vi "FL_Last_N_Samples_Cluster.vi"(1 "BufferLengthSamples":u32=20, 2 "Input cluster":T1) -> (0 "Output 1D array of clusters":cluster{"X":dbl, "Y":dbl}[](array[cluster]))   [LabVIEW 2016]
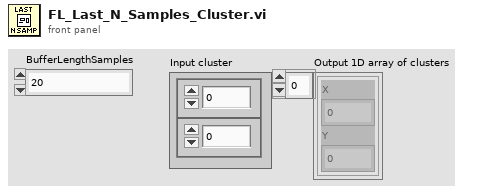
[diagram p1: front panel]
types:
  T1 = cluster{"Numeric Control":dbl, "Numeric Control":dbl}
  T2 = cluster{"Numeric Control":dbl, "Numeric Control":dbl}[]
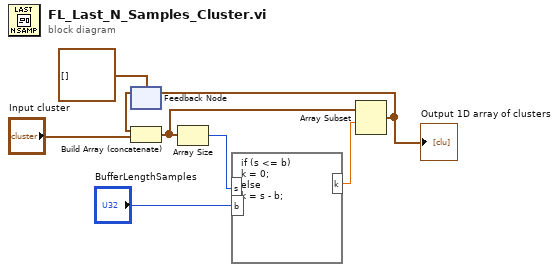
[diagram p0: block diagram]
diagram:
  n1 = feedback #1(T2 []) -> (w6:T2)
  n2 = Build Array (concatenate)(w6, "Input cluster") -> (w4:T2)
  n3 = Array Size(array=w4) -> (size(s)=w8:i32)
  n4 = formula code="if (s <= b)\nk = 0;\nelse\nk = s - b;"("s"=w8, "b"="BufferLengthSamples") -> ("k"=w7:dbl)
  n5 = Array Subset(array=w4, index=w7) -> (w3:T2)  [unwired: 1 in]
  "Output 1D array of clusters" <- w3
  n6 = feedback-in #1(w3) -> ()
